vi "Single DS Module.vi"(8 "error in (no error)":errorcluster caption="Error In", 11 "Queue":refnum<queue>) -> (0 "error out":errorcluster caption="Error Out")   [LabVIEW 2020]
uses:
  Save Type.ctl
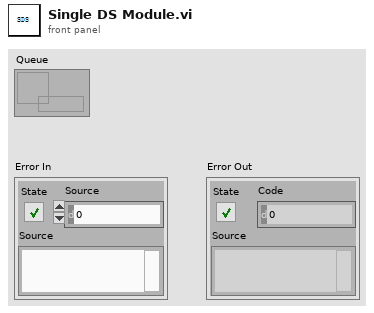
[diagram p1: front panel]
types:
  T1 = typedef "Save Type.ctl" = cluster{"Project":string, "Path":path, "Name":string, "Wave":waveform(sgl)}
  T2 = cluster{"Path":path, "tdmsRef":refnum<k34>, "QR":refnum<queue>, "Type":T1}
  T3 = enum16{"open", "open or create", "create or replace", "create", "open (read-only)"}
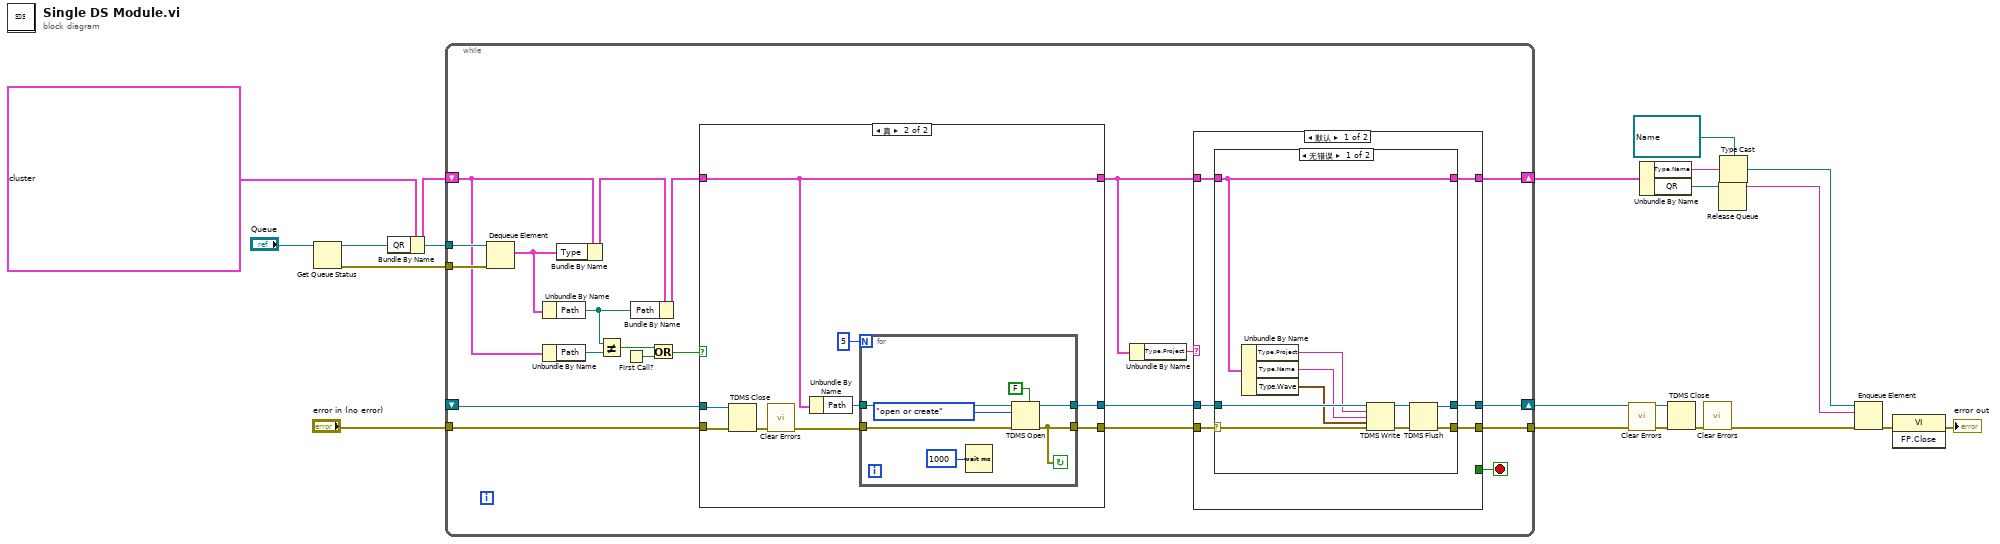
[diagram p0: block diagram]
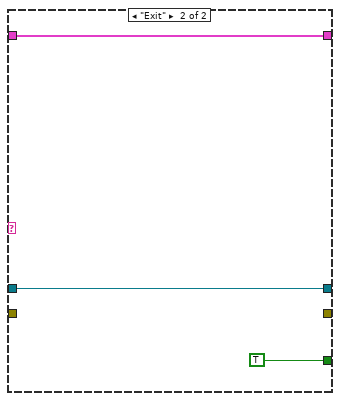
[diagram p3: hidden frame]
diagram:
  n1 = Get Queue Status(queue="Queue") -> (queue out=w3:refnum<queue>, error out=w5:errorcluster)  [unwired: 2 in, 6 out]
  n2 = Bundle By Name(cluster=T2 {"Path"=path "", "tdmsRef"=refnum, "QR"=refnum, "Type"={"Project"="", "Path"=path "", "Name"="", "Wave"={"t0"=timestamp(0 s since 1904-01-01), "dt"=1.0, "Y"=[]}}}, "QR"=w3) -> (w4:T2)
  n3 = while {
    tunnel: w3 -> [w40]
    tunnel: "error in (no error)" -> [w39]
    tunnel: [w35] -> w16
    shift-right: [w36] -> w17
    shift-left: _ -> [w34]
    shift-right: [w21] -> w2
    shift-left: w4 -> [w24]
    tunnel: w5 -> [w28]
    stop <- w33 stop-if-true
    n4 = Dequeue Element(queue=w40, error in (no error)=w28) -> (element=w27:T1)  [unwired: 1 in, 3 out]
    n5 = Unbundle By Name(w27) -> ("Path"=w22:path)
    n6 = Unbundle By Name(w24) -> ("Path"=w25:path)
    n7 = Bundle By Name(cluster=w24, "Type"=w27) -> (w26:T2)
    n8 = Not Equal?(x=w22, y=w25) -> (x != y?=w31:bool)
    n9 = First Call?() -> (First Call?: T/F=w30:bool)
    n10 = Bundle By Name(cluster=w26, "Path"=w22) -> (w23:T2)
    n11 = Or(x=w31, y=w30) -> (x .or. y?=w29:bool)
    n12 = case shown="真" w29 {
      tunnel: w39 -> [w64 w70]
      tunnel: [w63 w73] -> w38
      tunnel: [w64 w72] -> w37
      tunnel: w34 -> [w63 w68]
      tunnel: w23 -> [w62 w65]
      tunnel: [w62 w65] -> w20
      frame False {
      }
      frame True {
        n13 = TDMS Close(8:w70, 11:w68) -> (0:w69:errorcluster)  [unwired: 1 out]
        n14 = call <vilib>:"Clear Errors.vi"("error in (no error)"=w69) -> ("error out"=w67:errorcluster)  [unwired: 5 in, 1 out]
        n15 = Unbundle By Name(w65) -> ("Path"=w66:path)
        n16 = for {
          N: 5 -> [_]
          tunnel: [w78] -> w73
          tunnel: w66 -> [w77]
          tunnel: w67 -> [w79]
          tunnel: [w74] -> w72
          stop <- w74 continue-if-true
          n17 = Wait (ms)(milliseconds to wait=u32 1000 ("等待时间（毫秒）")) -> ()  [unwired: 1 out]
          n18 = TDMS Open(5:FALSE ("创建索引文件？(T)"), 8:w79, 10:T3."open or create" ("操作(0:open)"), 11:w77) -> (0:w74:errorcluster, 3:w78:refnum<k34>)  [unwired: 3 in]
        }
      }
    }
    n19 = Unbundle By Name(w20) -> ("Type.Project"=w32:string)
    n20 = case shown="默认" w32 {
      tunnel: w38 -> [w46 w61]
      tunnel: w37 -> [w45 _]
      tunnel: [w44 w61] -> w36
      tunnel: [w43 _] -> w35
      tunnel: [_ TRUE] -> w33
      tunnel: w20 -> [w42 w59]
      tunnel: [w41 w59] -> w21
      frame Default {
        n21 = case shown="无错误" w45 {
          selector: w45 -> [w55 _]
          tunnel: w46 -> [w56 w58]
          tunnel: [w48 w58] -> w44
          tunnel: [w50 _] -> w43
          tunnel: w42 -> [w47 w57]
          tunnel: [w47 w57] -> w41
          frame No Error {
            n22 = Unbundle By Name(w47) -> ("Type.Project"=w53:string, "Type.Name"=w52:string, "Type.Wave"=w51:waveform(sgl))
            n23 = TDMS Write(0:w56, 5:w53, 7:w52, 9:w51, 11:w55) -> (4:w49:refnum<k34>, 15:w54:errorcluster)  [unwired: 1 in, 2 out]
            n24 = TDMS Flush(4:w54, 7:w49) -> (0:w50:errorcluster, 3:w48:refnum<k34>)
          }
          frame Error {
          }
        }
      }
      frame "Exit" {
      }
    }
  }
  n25 = call <vilib>:"Clear Errors.vi"("error in (no error)"=w16) -> ("error out"=w10:errorcluster)  [unwired: 5 in, 1 out]
  n26 = Unbundle By Name(w2) -> ("Type.Name"=w15:string, "QR"=w1:refnum<queue>)
  n27 = TDMS Close(8:w10, 11:w17) -> (0:w9:errorcluster)  [unwired: 1 out]
  n28 = call <vilib>:"Clear Errors.vi"("error in (no error)"=w9) -> ("error out"=w8:errorcluster)  [unwired: 5 in, 1 out]
  n29 = Release Queue(queue=w1) -> (queue name=w12:string)  [unwired: 2 in, 2 out]
  n30 = Type Cast(type=refnum<queue> refnum ("queue out"), x=w15) -> (*(type *) &x=w13:refnum<queue>)
  n31 = Enqueue Element(queue=w13, element=w12, error in (no error)=w8) -> (error out=w19:errorcluster)  [unwired: 1 in, 2 out]
  n32 = invoke class="VI" method="FP.Close"(error in=w19) -> (error out=→"error out":errorcluster)  [unwired: 2 in, 2 out]
